vi "replace in NaN.vi"(11 "Data In":map{string, dbl}(c390)) -> (3 "Data Out":map{string, dbl}(c390))   [LabVIEW 2024, in "IOLink.lvlib"]
uses:
  IOLink.lvlib
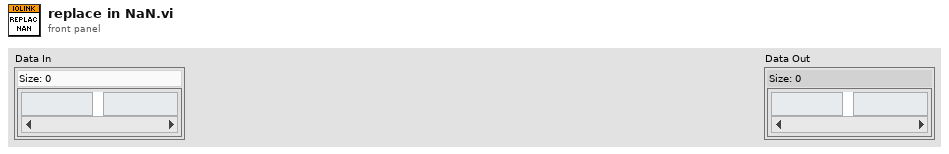
[diagram p1: front panel]
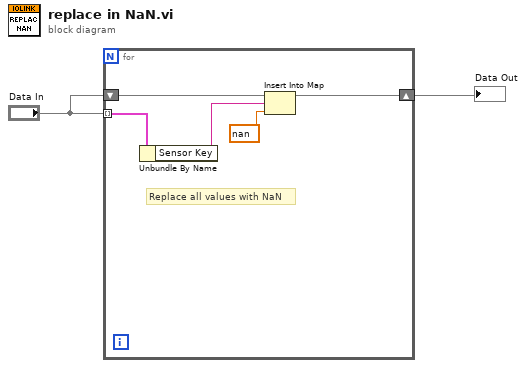
[diagram p0: block diagram]
diagram:
  n1 = for {
    tunnel: "Data In" -> [w7] mode=indexing
    shift-right: [w3] -> w1
    shift-left: "Data In" -> [w6]
    # "Replace all values with NaN"
    n2 = Unbundle By Name(w7) -> ("Sensor Key"=w5:string)
    n3 = Insert Into Map(map in=w6, key=w5, value=nan) -> (map out=w3:map{string, dbl})  [unwired: 2 out]
  }
  "Data Out" <- w1
